vi "Is Variant Supported Type.vi"(8 "error in (no error)":errorcluster, 11 "variant":variant) -> (0 "error out":errorcluster, 2 "Type":T1=enum."String", 3 "Is supported type?":bool)   [LabVIEW 2020, in "RxnRover.lvlib"]
doc: "Checks if the variant is any of the supported types for parameter values."
uses:
  RxnRover.lvlib
  Supported Parameter Variant Types.ctl
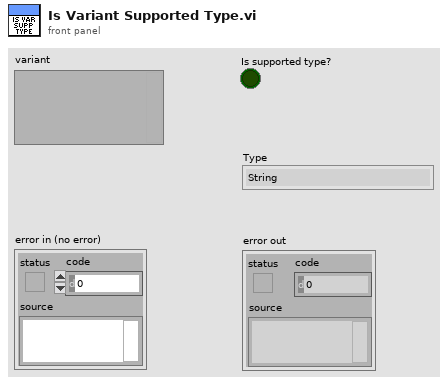
[diagram p1: front panel]
types:
  T1 = typedef "RxnRover.lvlib/Supported Parameter Variant Types.ctl" = enum16{"Unsupported", "Numeric", "Boolean", "String", "Path"}
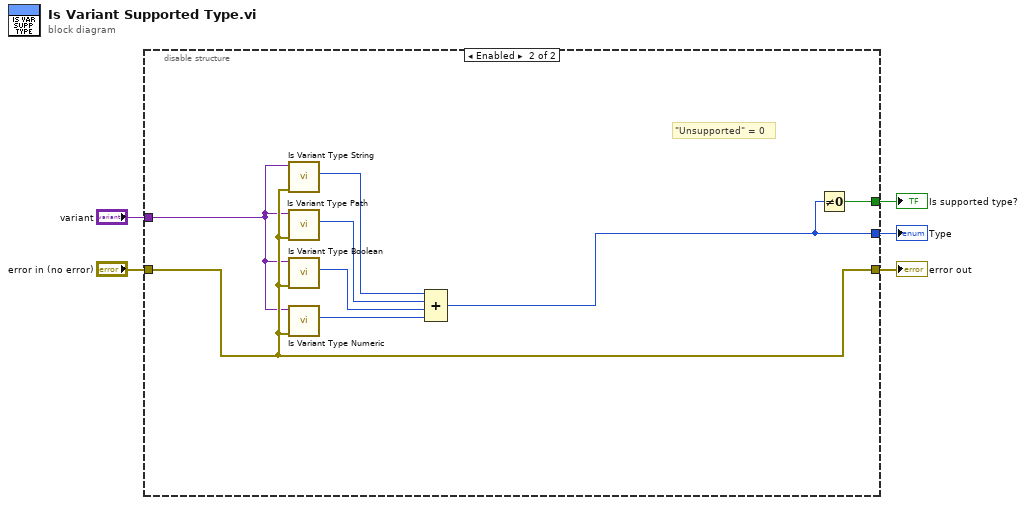
[diagram p0: block diagram]
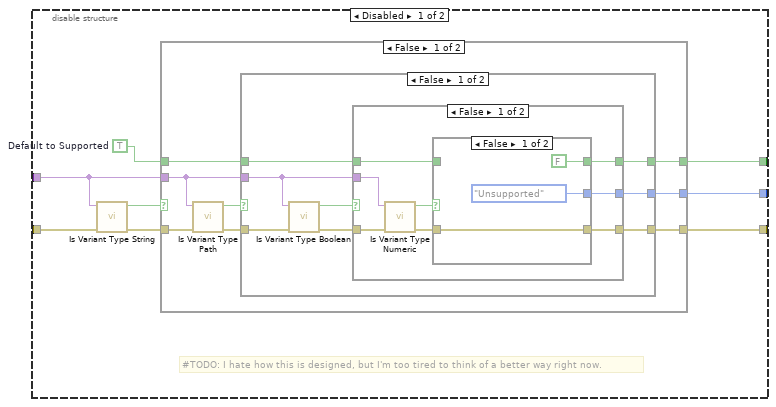
[diagram p2: hidden frame]
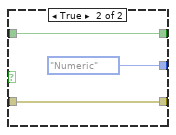
[diagram p3: hidden frame]
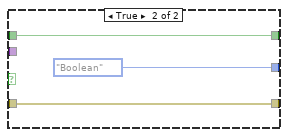
[diagram p4: hidden frame]
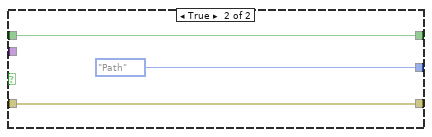
[diagram p5: hidden frame]
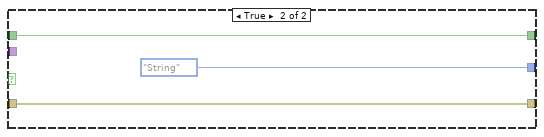
[diagram p6: hidden frame]
diagram:
  n1 = disable-structure shown="Enabled" {
    disable-tunnel: "error in (no error)" -> [w13 w60]
    disable-tunnel: [w12 w60] -> w4
    disable-tunnel: [w9 w54] -> w3
    disable-tunnel: "variant" -> [w8 w53]
    disable-tunnel: [w7 w55] -> w1
    frame Disabled {
      w6 = TRUE  # Default to Supported
      # "#TODO: I hate how this is designed, but I'm too tired to think of a better way right now."
      n2 = call "Is Variant Type String.vi"("error in (no error)"=w13, "variant"=w8) -> ("error out"=w11:errorcluster, "Is string?"=w10:bool)  [unwired: 7 in, 1 out]
      n3 = case shown="False" w10 {
        tunnel: [w21 w52] -> w12
        tunnel: w11 -> [w20 w52]
        tunnel: [w16 Supported_Parameter_Variant_Types."String" ("Supported Parameter Variant Types")] -> w9
        tunnel: w8 -> [w17 _]
        tunnel: w6 -> [w15 w50]
        tunnel: [w14 w50] -> w7
        frame False {
          n4 = call "Is Variant Type Path.vi"("error in (no error)"=w20, "variant"=w17) -> ("error out"=w19:errorcluster, "Is path?"=w18:bool)  [unwired: 7 in, 1 out]
          n5 = case shown="False" w18 {
            tunnel: [w29 w48] -> w21
            tunnel: w19 -> [w28 w48]
            tunnel: w17 -> [w25 _]
            tunnel: [w24 Supported_Parameter_Variant_Types."Path" ("Supported Parameter Variant Types")] -> w16
            tunnel: w15 -> [w23 w47]
            tunnel: [w22 w47] -> w14
            frame False {
              n6 = call "Is Variant Type Boolean.vi"("error in (no error)"=w28, "variant"=w25) -> ("error out"=w27:errorcluster, "Is boolean?"=w26:bool)  [unwired: 7 in, 1 out]
              n7 = case shown="False" w26 {
                tunnel: [w33 w46] -> w29
                tunnel: w27 -> [w37 w46]
                tunnel: w25 -> [w36 _]
                tunnel: [w32 Supported_Parameter_Variant_Types."Boolean" ("Supported Parameter Variant Types")] -> w24
                tunnel: w23 -> [w31 w44]
                tunnel: [w30 w44] -> w22
                frame False {
                  n8 = call "Is Variant Type Numeric.vi"("error in (no error)"=w37, "variant"=w36) -> ("error out"=w34:errorcluster, "Is numeric?"=w35:bool)  [unwired: 7 in, 1 out]
                  n9 = case shown="False" w35 {
                    tunnel: w34 -> [w40 w43]
                    tunnel: [w40 w43] -> w33
                    tunnel: [Supported_Parameter_Variant_Types."Unsupported" ("Supported Parameter Variant Types") Supported_Parameter_Variant_Types."Numeric" ("Supported Parameter Variant Types")] -> w32
                    tunnel: w31 -> [_ w41]
                    tunnel: [FALSE ("Default to Supported") w41] -> w30
                    frame False {
                    }
                    frame True {
                    }
                  }
                }
                frame True {
                }
              }
            }
            frame True {
            }
          }
        }
        frame True {
        }
      }
    }
    frame Enabled {
      # "\"Unsupported\" = 0"
      n10 = call "Is Variant Type String.vi"("error in (no error)"=w60, "variant"=w53) -> ("Type"=w59:T1)  [unwired: 7 in, 2 out]
      n11 = call "Is Variant Type Path.vi"("error in (no error)"=w60, "variant"=w53) -> ("Type"=w58:T1)  [unwired: 7 in, 2 out]
      n12 = call "Is Variant Type Boolean.vi"("error in (no error)"=w60, "variant"=w53) -> ("Type"=w57:T1)  [unwired: 7 in, 2 out]
      n13 = call "Is Variant Type Numeric.vi"("error in (no error)"=w60, "variant"=w53) -> ("Type"=w56:T1)  [unwired: 7 in, 2 out]
      n14 = Compound Arithmetic op=unknown(w59, w58, w57, w56) -> (w54:u16)
      n15 = Not Equal To 0?(x=w54) -> (x != 0?=w55:bool)
    }
  }
  "error out" <- w4
  "Type" <- w3
  "Is supported type?" <- w1
